vi "Create Session.vi"(5 "Session in":refnum<class "Session.lvclass">, 6 "Type":T1, 7 "Close Session":refnum<user-event>, 8 "error in (no error)":errorcluster, 9 "Request":refnum<queue>, 10 "Keep Alive (s)":i32, 11 "Connection":refnum<class "TCPConnection.lvclass">) -> (0 "error out":errorcluster, 3 "Session":refnum<class "Session.lvclass">)   [LabVIEW 2013, in "MQTT Server.lvlib" / "Session.lvclass"]
uses:
  Session.lvclass
  Connection/TCPConnection.lvclass
  MQTT_Base/Request -- cluster.ctl
  Control Packets/ControlPacket/ControlPacket.lvclass
  MQTT_Base/Response -- cluster.ctl
  Session Type -- enum.ctl
  Session State -- cluster.ctl
  Control Packets/SUBSCRIBE/Topic Subscription -- cluster.ctl
  Control Packets/ControlPacket/QualityOfService -- enum.ctl
  Control Packets/ControlPacket/Pending Transmission -- cluster.ctl
  Pending ACKs -- cluster.ctl
  Session.lvclass/Session.ctl
  MQTT_Base/MQTT_Base.lvclass
  Control Packets/SUBSCRIBE/SUBSCRIBE.lvclass
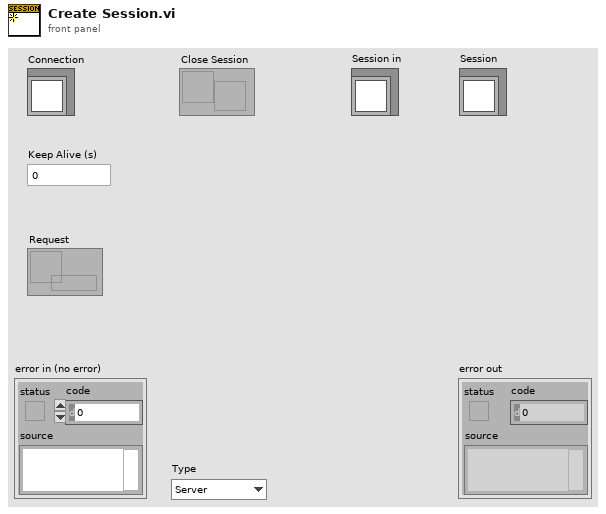
[diagram p1: front panel]
types:
  T1 = typedef "MQTT Server.lvlib/Session.lvclass/Session Type -- enum.ctl" = enum16{"Server", "Client"}
  T2 = typedef "MQTT Server.lvlib/MQTT_Base.lvclass/Response -- cluster.ctl" = cluster{"Packet":refnum<class "ControlPacket.lvclass">, "Protocol Error":errorcluster, "disconnect session":bool, "[ACK]":refnum<notifier>[]}
  T3 = typedef "MQTT Server.lvlib/Session.lvclass/Session State -- cluster.ctl" = cluster{"CleanSession":bool, "Client ID":string, "Subscriptions":T4[], "Pending Transmissions":T6[], "Pending ACKs":T7[]}
  T4 = typedef "SUBSCRIBE.lvclass/Topic Subscription -- cluster.ctl" = cluster{"Topic Filter":string, "QoS":T5}
  T5 = typedef "ControlPacket.lvclass/QualityOfService -- enum.ctl" = enum16{"0 (At Most Once)", "1 (At Least Once)", "2 (Exactly Once)"}
  T6 = typedef "ControlPacket.lvclass/Pending Transmission -- cluster.ctl" = cluster{"Message":refnum<class "ControlPacket.lvclass">, "QoS":T5, "Tx-Rx":bool}
  T7 = typedef "MQTT Server.lvlib/Session.lvclass/Pending ACKs -- cluster.ctl" = cluster{"Message":refnum<class "ControlPacket.lvclass">, "[ACK]":refnum<notifier>[], "Packet Identifier":u16}
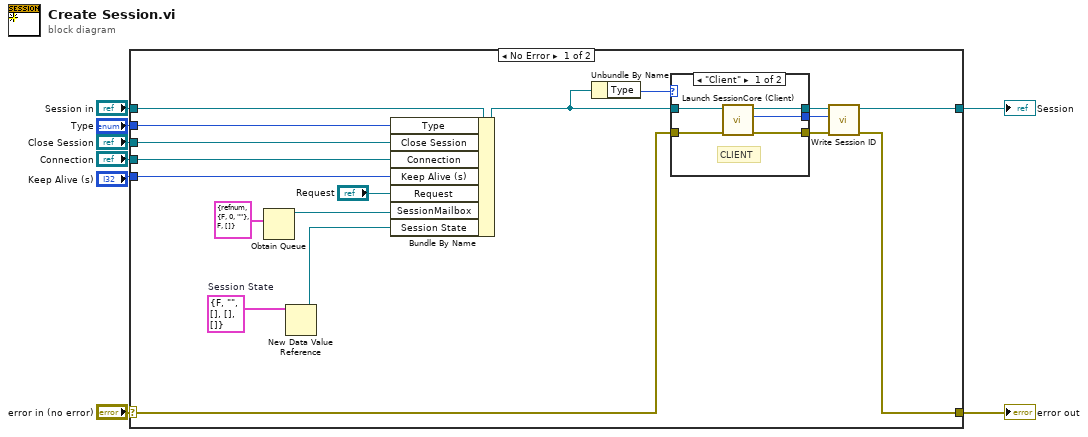
[diagram p0: block diagram]
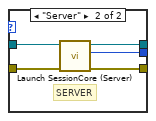
[diagram p2: hidden frame]
diagram:
  n1 = case shown="No Error" "error in (no error)" {
    selector: "error in (no error)" -> [w19 w37]
    tunnel: [w12 w37] -> w7
    tunnel: [w18 w36] -> w5
    tunnel: "Session in" -> [w24 w36]
    tunnel: "Keep Alive (s)" -> [w22 _]
    tunnel: "Connection" -> [w21 _]
    tunnel: "Close Session" -> [w17 _]
    tunnel: "Type" -> [w11 _]
    frame No Error {
      w16 = T3 {"CleanSession"=FALSE, "Client ID"="", "Subscriptions"=[], "Pending Transmissions"=[], "Pending ACKs"=[]}  # Session State
      n2 = Obtain Queue(element data type=T2 {"Packet"=refnum, "Protocol Error"={"status"=FALSE, "code"=0, "source"=""}, "disconnect session"=FALSE, "[ACK]"=[]} ("Response")) -> (queue out=w25:refnum<queue>)  [unwired: 4 in, 2 out]
      n3 = New Data Value Reference(data value=w16) -> (data value reference=w15:refnum<data-value>)  [unwired: 1 in, 1 out]
      n4 = Bundle By Name(cluster=w24, "Type"=w11, "Close Session"=w17, "Connection"=w21, "Keep Alive (s)"=w22, "Request"="Request", "SessionMailbox"=w25, "Session State"=w15) -> (w10:refnum<class "Session.lvclass">)
      n5 = Unbundle By Name(w10) -> ("Type"=w9:T1)
      n6 = case shown="\"Client\"" w9 {
        tunnel: w19 -> [w29 w35]
        tunnel: [w27 w34] -> w14
        tunnel: w10 -> [w30 w33]
        tunnel: [w28 w32] -> w13
        tunnel: [w26 w31] -> w12
        frame "Client" {
          # "CLIENT"
          n7 = call "Launch SessionCore (Client).vi"("error in (no error)"=w29, "Session in"=w30) -> ("error out"=w26:errorcluster, "Session ID"=w27:i32, "Session out"=w28:refnum<class "Session.lvclass">)  [unwired: 7 in]
        }
        frame "Server" {
          # "SERVER"
          n8 = call "Launch SessionCore (Server).vi"("error in (no error)"=w35, "Session in"=w33) -> ("error out"=w31:errorcluster, "Session ID"=w34:i32, "Session out"=w32:refnum<class "Session.lvclass">)  [unwired: 7 in]
        }
      }
      n9 = call "Write Session ID.vi"("Session ID"=w14, "Session in"=w13) -> ("Session out"=w18:refnum<class "Session.lvclass">)  [unwired: 8 in, 1 out]
    }
    frame Error {
    }
  }
  "error out" <- w7
  "Session" <- w5
